vi "DMM Scan Reset_3.vi"(11 "VISA in resource name":refnum<visa-resource-name>) -> (0 "error out":errorcluster, 3 "VISA resource name out":refnum<visa-resource-name>)   [LabVIEW 2023]
uses:
  <instrlib>/Agilent 3446X Series/Agilent 3446X Series.lvlib
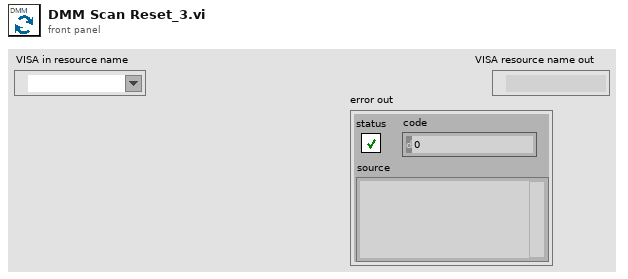
[diagram p1: front panel]
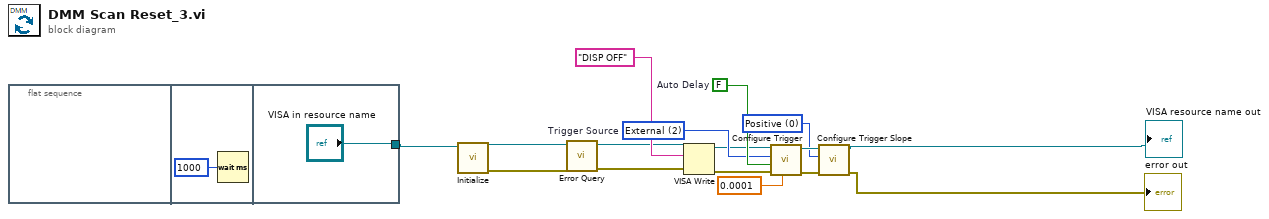
[diagram p0: block diagram]
diagram:
  w14 = 0 items=["Positive", "Negative"] ("Trigger Edge (1: Negative)")
  w12 = 2 items=["Immediate", "Software (Bus)", "External"]  # Trigger Source
  w13 = FALSE  # Auto Delay
  n1 = flat-sequence {
    tunnel: ["VISA in resource name"] -> w3
    frame #0 {
    }
    frame #1 {
      n2 = Wait (ms)(milliseconds to wait=u32 1000) -> ()  [unwired: 1 out]
    }
    frame #2 {
    }
  }
  n3 = call <instrlib>:"Initialize.vi"("VISA resource name"=w3) -> ("error out"=w5:errorcluster, "VISA resource name out"=w4:refnum<visa-resource-name>)  [unwired: 4 in, 5 out]
  n4 = call <instrlib>:"Error Query.vi"("error in (no error)"=w5, "VISA resource name"=w4) -> ("error out"=w6:errorcluster, "VISA resource name out"=w7:refnum<visa-resource-name>)  [unwired: 8 out]
  n5 = VISA Write(VISA resource name=w7, write buffer="DISP OFF", error in (no error)=w6) -> (VISA resource name out=w9:refnum<visa-resource-name>, error out=w8:errorcluster)  [unwired: 1 out]
  n6 = call <instrlib>:"Configure Trigger.vi"("Manual Trigger Delay (1 s)"=0.0001, "error in (no error)"=w8, "Auto Delay (F:Disable)"=w13, "Trigger Source (0: Immediate)"=w12, "VISA resource name"=w9) -> ("error out"=w16:errorcluster, "VISA resource name out"=w15:refnum<visa-resource-name>)  [unwired: 1 in, 4 out]
  n7 = call <instrlib>:"Configure Trigger Slope.vi"("error in (no error)"=w16, "Trigger Edge (1: Negative)"=w14, "VISA resource name"=w15) -> ("error out"=→"error out":errorcluster, "VISA resource name out"=→"VISA resource name out":refnum<visa-resource-name>)  [unwired: 7 in]
